vi "SetVelocity.vi"() -> ()   [LabVIEW 2011]
uses:
  Robot Global Data.vi
  <vilib>/addons/control/pid/pid.llb/PID (DBL).vi
  <vilib>/addons/control/pid/NI_PID_pid.lvlib
panel:
  out "Waveform Chart":dbl(graph)
  out "RPM":dbl
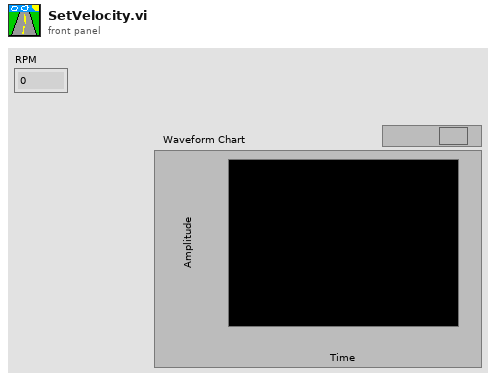
[diagram p1: front panel]
types:
  T1 = typedef "WPI_MotorControlDeviceRef.ctl" = cluster{"DeviceStatus":errorcluster, "Type":enum16{"PWM", "CAN"}, "PWM":cluster{"Digital Module":T2, "PWM Channel":T3, "DeadBand":T4}, "CAN":cluster{"Device Number":u8, "Control Mode":T5, "Semaphore":T6, "Max Vout":dbl}, "Invert":bool, "TransformRef":T7, "InvTransformRef":T7}
  T2 = typedef "FPGA_TypedefDigitalModule.ctl" = enum16{"Digital Module 1", "Digital Module 2"}
  T3 = typedef "FPGA_DIOPWMChannel.ctl" = enum8{"PWM 1", "PWM 2", "PWM 3", "PWM 4", "PWM 5", "PWM 6", "PWM 7", "PWM 8", "PWM 9", "PWM 10", "Invalid"}
  T4 = typedef "WPI_PWMDeadband.ctl" = cluster{"Name":string, "maxPositivePwm":i32, "minPositivePwm":i32, "centerPwm":i32, "maxNegativePwm":i32, "minNegativePwm":i32, "angularRange":u16}
  T5 = typedef "WPI_CANJaguar_ControlMode.ctl" = enum8{"Percent VBus", "Current", "Speed", "Position", "Voltage"}
  T6 = typedef "Semaphore RefNum" = refnum<k1>
  T7 = typedef "WPI_PWMTransform_ConPane.ctl" = refnum<vi>
  T8 = cluster{"proportional gain (Kc)":dbl, "integral time (Ti, min)":dbl, "derivative time (Td, min)":dbl}
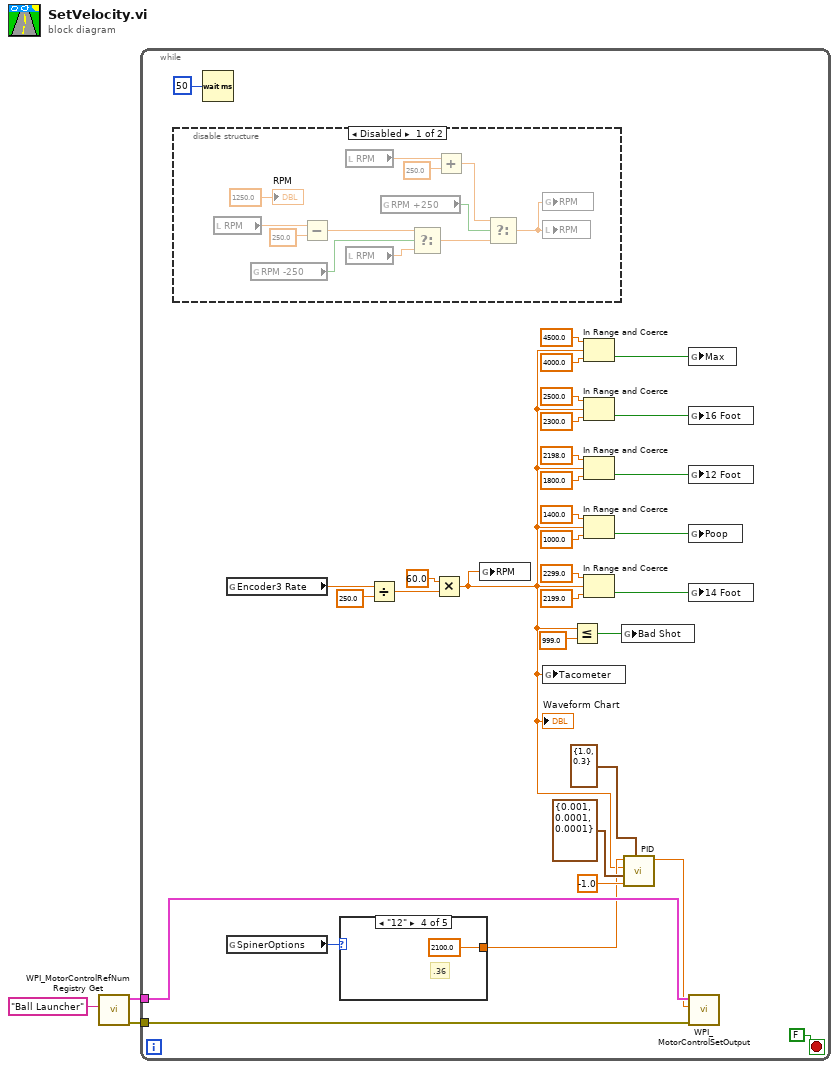
[diagram p0: block diagram]
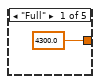
[diagram p2: hidden frame]
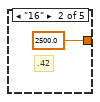
[diagram p3: hidden frame]
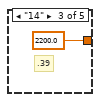
[diagram p4: hidden frame]
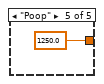
[diagram p5: hidden frame]
diagram:
  n1 = call <vilib>:"WPI_MotorControlRefNum Registry Get.vi"("refnum name"="Ball Launcher") -> ("error out"=w1:errorcluster, "MotorControlDevRef"=w2:T1)  [unwired: 9 in]
  n2 = while {
    tunnel: w2 -> [w35]
    tunnel: w1 -> [w34]
    stop <- FALSE stop-if-true
    n3 = disable-structure shown="Disabled" {
      frame Disabled {
        n4 = local read "RPM"() -> (w43:dbl)
        n5 = global read "Robot Global Data.vi" "RPM -250"() -> (w49:bool)
        n6 = Subtract(x=w43, y=250.0) -> (x-y=w48:dbl)
        n7 = local read "RPM"() -> (w45:dbl)
        n8 = local read "RPM"() -> (w44:dbl)
        n9 = global read "Robot Global Data.vi" "RPM +250"() -> (w52:bool)
        n10 = Select(t=w48, s=w49, f=w44) -> (s? t:f=w47:dbl)
        n11 = Add(x=w45, y=250.0) -> (x+y=w51:dbl)
        n12 = Select(t=w51, s=w52, f=w47) -> (s? t:f=w42:dbl)
        n13 = global write "Robot Global Data.vi" "RPM"(w42) -> ()
        n14 = local write "RPM"(w42) -> ()
        "RPM" <- 1250.0 ("RPM")
      }
      frame Enabled {
      }
    }
    n15 = Wait (ms)(milliseconds to wait=50) -> ()  [unwired: 1 out]
    n16 = global read "Robot Global Data.vi" "Encoder3 Rate"() -> (w28:dbl)
    n17 = global read "Robot Global Data.vi" "SpinerOptions"() -> (w7:enum16{"Full", "16", "14", "12", "Poop"})
    n18 = case shown="\"12\"" w7 {
      tunnel: [4300.0 2500.0 2200.0 2100.0 1250.0] -> w6
      frame "Full" {
      }
      frame "16" {
        # ".42"
      }
      frame "14" {
        # ".39"
      }
      frame "12" {
        # ".36"
      }
      frame "Poop" {
      }
    }
    n19 = Divide(x=w28, y=250.0) -> (x/y=w26:dbl)
    n20 = Multiply(x=60.0, y=w26) -> (x*y=w4:dbl)
    "Waveform Chart" <- w4
    n21 = global write "Robot Global Data.vi" "RPM"(w4) -> ()
    n22 = global write "Robot Global Data.vi" "Tacometer"(w4) -> ()
    n23 = Less Or Equal?(x=w4, y=999.0) -> (x <= y?=w8:bool)
    n24 = In Range and Coerce(upper limit=4500.0, x=w4, lower limit=4000.0) -> (In Range?=w9:bool)  [unwired: 1 out]
    n25 = In Range and Coerce(upper limit=2500.0, x=w4, lower limit=2300.0) -> (In Range?=w10:bool)  [unwired: 1 out]
    n26 = In Range and Coerce(upper limit=2198.0, x=w4, lower limit=1800.0) -> (In Range?=w12:bool)  [unwired: 1 out]
    n27 = In Range and Coerce(upper limit=1400.0, x=w4, lower limit=1000.0) -> (In Range?=w13:bool)  [unwired: 1 out]
    n28 = In Range and Coerce(upper limit=2299.0, x=w4, lower limit=2199.0) -> (In Range?=w11:bool)  [unwired: 1 out]
    n29 = global write "Robot Global Data.vi" "Bad Shot"(w8) -> ()
    n30 = call-poly <vilib>:"PID.vi"("output range"=cluster{"output high":dbl, "output low":dbl} {"output high"=1.0, "output low"=0.3}, "dt (s)"=-1.0, "PID gains"=T8 {"proportional gain (Kc)"=0.001, "integral time (Ti, min)"=0.0001, "derivative time (Td, min)"=0.0001}, "process variable"=w4, "setpoint"=w6) -> ("output"=w5:dbl)  [unwired: 5 in, 1 out]
    n31 = global write "Robot Global Data.vi" "Max"(w9) -> ()
    n32 = global write "Robot Global Data.vi" "16 Foot"(w10) -> ()
    n33 = global write "Robot Global Data.vi" "12 Foot"(w12) -> ()
    n34 = global write "Robot Global Data.vi" "Poop"(w13) -> ()
    n35 = global write "Robot Global Data.vi" "14 Foot"(w11) -> ()
    n36 = call <vilib>:"WPI_MotorControlSetOutput.vi"("error in (no error)"=w34, "Output"=w5, "MotorControlDevRef"=w35) -> ()  [unwired: 7 in, 2 out]
  }
